vi "Add Module to Project by Path.vi"(6 "TreeControl in":refnum<vi>, 8 "error in":errorcluster, 9 "Module Name":string, 10 "Module Folder":path, 11 "Project":refnum<class "Project.lvclass">) -> (0 "error out":errorcluster, 3 "Project Out":refnum<class "Project.lvclass">)   [LabVIEW 2019, in "Panther Dashboard.lvlib"]
doc: "Gets the Singleton and Cloneable references and creates a list of each type of DQMH Modules"
uses:
  Panther Dashboard.lvlib
  Class/Project/Project.lvclass
  Class/Library/Library.lvclass
  C:/GitClones/PantherDashboard/src/LabVIEW/Panther Dashboard/Class/LabVIEWItem/LabVIEWItem.lvclass
  Module type--enum.ctl
  Class/Project/Project.lvclass/Project.ctl
  Class/Library/Library.lvclass/Library.ctl
  Class/LabVIEWItem/LabVIEWItem.lvclass/LabVIEWItem.ctl
  Class/Project/Read Target App Ins Ref.vi
  Class/Library/Write Library Ref.vi
  Class/LabVIEWItem/Write Item Name.vi
  Class/LabVIEWItem/Write Item Description.vi
  Class/LabVIEWItem/Write Item Path.vi
  Class/Library/Write Type.vi
  Class/LabVIEWItem/Read Item Name.vi
  Class/Project/Read Libraries.vi
  Class/Project/Write Libraries.vi
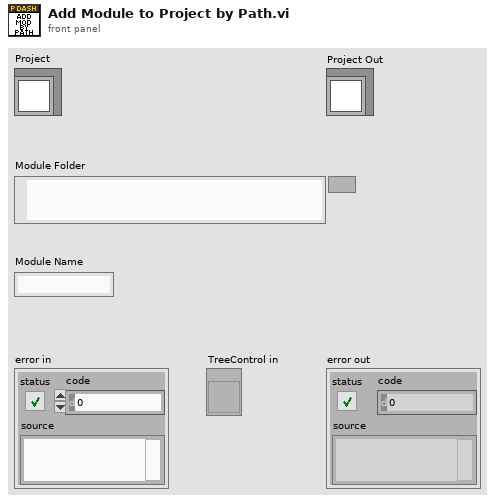
[diagram p1: front panel]
types:
  T1 = typedef "Panther Dashboard.lvlib/Module type--enum.ctl" = enum16{"Singleton", "Cloneable"}
  T2 = typedef "Tree Map.lvlib/Tree Map Data.ctl" = map{string, cluster{"Child Paths Set":set{string}, "Name":string, "Data":string, "Attributes":map{string, string}}}
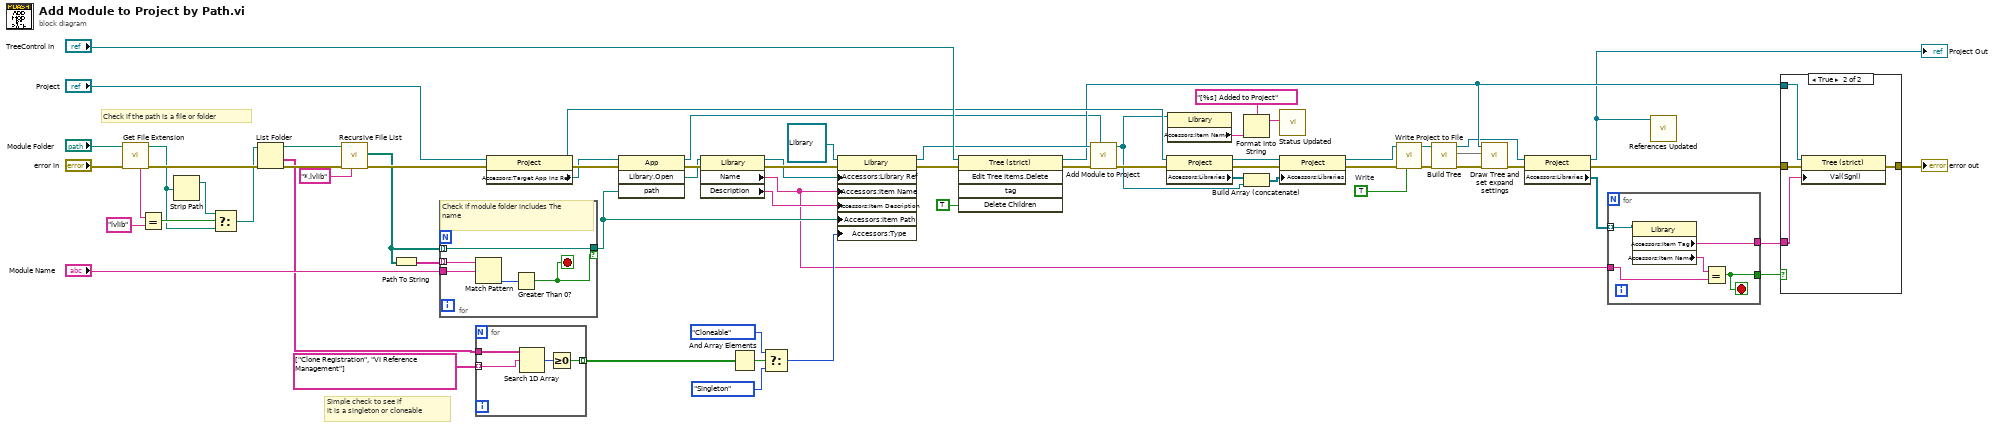
[diagram p0: block diagram]
diagram:
  w45 = TRUE  # Write
  # "Check if the path is a file or folder"
  # "Simple check to see if\nit is a singleton or cloneable"
  n1 = call <vilib>:"Get File Extension.vi"("error in (no error)"="error in", "file"="Module Folder") -> ("error out"=w13:errorcluster, "dup file"=w8:path, "unmodified file extension"=w12:string)  [unwired: 5 in, 2 out]
  n2 = Equal?(x=w12, y="lvlib") -> (x = y?=w10:bool)
  n3 = Strip Path(path=w8) -> (stripped path=w7:path)  [unwired: 1 out]
  n4 = Select(t=w7, s=w10, f=w8) -> (s? t:f=w9:path)
  n5 = List Folder(path=w9, error in=w13) -> (path out=w17:path, folder names=w24:string[], error out=w54:errorcluster)  [unwired: 2 in, 1 out]
  n6 = call <vilib>:"Recursive File List.vi"("pattern"="*.lvlib", "error in (no error)"=w54, "Folder Path"=w17) -> ("error out"=w53:errorcluster, "All Files in Dir"=w30:path[])  [unwired: 4 in, 3 out]
  n7 = Path To String(path=w30) -> (string=w32:string[])
  n8 = for {
    tunnel: w32 -> [w71] mode=indexing
    tunnel: "Module Name" -> [w70]
    tunnel: w30 -> [w69] mode=indexing
    tunnel: [w69] -> w25 if=w67
    stop <- w67 stop-if-true
    # "Check if module folder includes The name"
    n9 = Match Pattern(string=w71, regular expression=w70) -> (offset past match=w68:i32)  [unwired: 1 in, 3 out]
    n10 = Greater Than 0?(x=w68) -> (x > 0?=w67:bool)
  }
  n11 = for {
    tunnel: w24 -> [w75]
    tunnel: string[] ["Clone Registration", "VI Reference Management"] ("folder names") -> [w74] mode=indexing
    tunnel: [w72] -> w22 mode=indexing
    n12 = Search 1D Array(1D array=w75, element=w74) -> (index of element=w73:i32)  [unwired: 1 in]
    n13 = Greater Or Equal To 0?(x=w73) -> (x >= 0?=w72:bool)
  }
  n14 = property class="Project"(reference="Project", error in=w53) -> (reference out=w49:refnum<class "Project.lvclass">, error out=w52:errorcluster, "Accessors:Target App Ins Ref"=w29:refnum<vi>)
  n15 = invoke class="App" method="Library.Open"(reference=w29, error in=w52, "path"=w25) -> (reference out=w16:refnum<vi>, error out=w56:errorcluster, "Open Library"=w28:refnum<vi>)  [unwired: 1 in, 1 out]
  n16 = property class="Library"(reference=w28, error in=w56) -> (reference out=w27:refnum<vi>, error out=w55:errorcluster, "Name"=w3:string, "Description"=w26:string)
  n17 = And Array Elements(Boolean array=w22) -> (logical AND=w19:bool)
  n18 = Select(t=Module_type--enum."Cloneable", s=w19, f=Module_type--enum."Singleton" ("Type")) -> (s? t:f=w20:T1)
  n19 = property class="Library"(reference=refnum<class "Library.lvclass"> refnum ("Panther Dashboard.lvlib:Library"), error in=w55, "Accessors:Library Ref"=w27, "Accessors:Item Name"=w3, "Accessors:Item Description"=w26, "Accessors:Item Path"=w25, "Accessors:Type"=w20) -> (reference out=w47:refnum<class "Library.lvclass">, error out=w57:errorcluster)
  n20 = invoke class="Tree (strict)" method="Edit Tree Items.Delete"(reference="TreeControl in", error in=w57, "Delete Children"=TRUE ("Delete Children?")) -> (reference out=w39:refnum<vi>, error out=w60:errorcluster)  [unwired: 2 in, 3 out]
  n21 = call "Add Module to Project.vi"("App Ref"=w16, "error in"=w60, "Library In"=w47) -> ("error out"=w63:errorcluster, "Library Out"=w35:refnum<class "Library.lvclass">)  [unwired: 7 in]
  n22 = property class="Project"(reference=w49, error in=w63) -> (reference out=w42:refnum<class "Project.lvclass">, error out=w62:errorcluster, "Accessors:Libraries"=w44:refnum<class "Library.lvclass">[])
  n23 = property class="Library"(reference=w35) -> ("Accessors:Item Name"=w34:string)  [unwired: 1 in, 2 out]
  n24 = Format Into String(format string="[%s] Added to Project" ("Status"), w34) -> (resulting string=w36:string)  [unwired: 2 in, 1 out]
  n25 = Build Array (concatenate)(w44, w35) -> (w43:refnum<class "Library.lvclass">[])
  n26 = call "Status Updated.vi"("Status"=w36) -> ()  [unwired: 10 in, 1 out]
  n27 = property class="Project"(reference=w42, error in=w62, "Accessors:Libraries"=w43) -> (reference out=w41:refnum<class "Project.lvclass">, error out=w61:errorcluster)
  n28 = call "Write Project to File.vi"("Write"=w45, "error in"=w61, "Project In"=w41) -> ("error out"=w65:errorcluster, "Project Out"=w38:refnum<class "Project.lvclass">)  [unwired: 6 in, 1 out]
  n29 = call "Build Tree.vi"("error in"=w65, "Project in"=w38) -> ("error out"=w64:errorcluster, "Tree Map Out"=w40:T2, "Project Out"=w6:refnum<class "Project.lvclass">)  [unwired: 7 in]
  n30 = call "Draw Tree and set expand settings.vi"("error in"=w64, "Tree Map In"=w40, "TreeControl in"=w39) -> ("error out"=w59:errorcluster)  [unwired: 8 in]
  n31 = property class="Project"(reference=w6, error in=w59) -> (reference out=w5:refnum<class "Project.lvclass">, error out=w58:errorcluster, "Accessors:Libraries"=w4:refnum<class "Library.lvclass">[])
  "Project Out" <- w5
  n32 = for {
    tunnel: w4 -> [w80] mode=indexing
    tunnel: w3 -> [w78]
    tunnel: [w77] -> w2
    tunnel: [w76] -> w1
    stop <- w76 stop-if-true
    n33 = property class="Library"(reference=w80) -> ("Accessors:Item Tag"=w77:string, "Accessors:Item Name"=w79:string)  [unwired: 1 in, 2 out]
    n34 = Equal?(x=w79, y=w78) -> (x = y?=w76:bool)
  }
  n35 = call "References Updated.vi"("Project"=w5) -> ()  [unwired: 10 in, 1 out]
  n36 = case shown="True" w1 {
    tunnel: [w81 w85] -> w66
    tunnel: w58 -> [w81 w84]
    tunnel: w39 -> [_ w83]
    tunnel: w2 -> [_ w82]
    frame False {
    }
    frame True {
      n37 = property class="Tree (strict)"(reference=w83, error in=w84, "Val(Sgnl)"=w82) -> (error out=w85:errorcluster)  [unwired: 1 out]
    }
  }
  "error out" <- w66
